vi "midiInStop.vi"(8 "error in":errorcluster, 11 "midi in":refnum<class "midi.lvclass">) -> (0 "error out":errorcluster, 3 "midi out":refnum<class "midi.lvclass">)   [LabVIEW 2020, in "midi.lvclass"]
doc: "The midiInStop function stops MIDI input on the specified MIDI input device.\n\nIf there are any system-exclusive messages or stream buffers in the queue, the current buffer is marked as done (the dwBytesRecorded member of the MIDIHDR structure will contain the actual length of data), but any empty buffers in the queue remain there and are not marked as done. Calling this function when input is not started has no effect, and the function returns zero."
uses:
  midi.lvclass
  midi.lvclass/midi.ctl
  cpp-src/MIDIInToLabVIEWWrapper/x64/Release/MIDIInToLabVIEWWrapper.dll
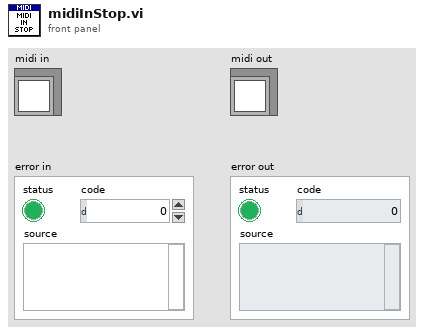
[diagram p1: front panel]
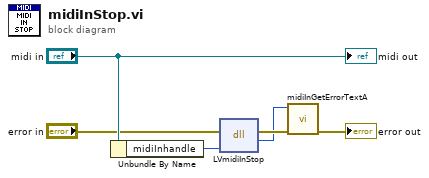
[diagram p0: block diagram]
diagram:
  n1 = Unbundle By Name("midi in") -> ("midiInhandle"=w4:u64)
  n2 = dll-call lib="C:/code/LabVIEW-MIDI/cpp-src/MIDIInToLabVIEWWrapper/x64/Release/MIDIInToLabVIEWWrapper.dll" fn="LVmidiInStop"(error in="error in", "hMidiIn"=w4) -> (error out=w2:errorcluster, "error"=w1:i32)  [unwired: 3 in, 1 out]
  n3 = call "midiInGetErrorTextA.vi"("error in"=w2, "Error Code"=w1) -> ("error out"=→"error out":errorcluster)  [unwired: 9 in]
  "midi out" <- "midi in"
